vi "PH_BL-Master.PC _6P 4Q Position.vi"(0 "i ref in":refnum<vi>, 2 "6P 4Q Instance":string, 3 "Selector":T1 items=["unknown", "Position I", "Position II", "Position III", "Position IV", "moving"], 4 "no Link":bool, 5 "error in (no error)":errorcluster) -> (14 "i ref out":refnum<vi>, 19 "error out":errorcluster)   [LabVIEW 2014, in "PH_BL-Master.lvlib"]
doc: "This VI writes the incoming information to own attributes."
uses:
  PH_BL-Master.lvlib
  PH_Motion/PH_4_Pos_Selector/PH_4_Pos_Selector.Position Selector.ctl
  PH_Motion/PH_4_Pos_Selector/PH_4_Pos_Selector.lvlib
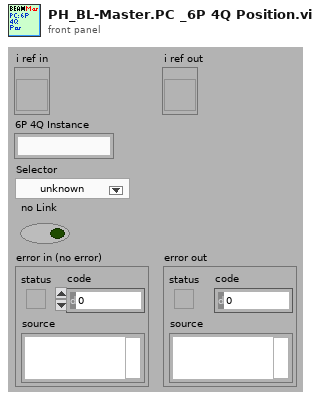
[diagram p1: front panel]
types:
  T1 = typedef "PH_4_Pos_Selector.lvlib/PH_4_Pos_Selector.Position Selector.ctl" = u16
  T2 = typedef "PH_BL-Master.lvlib/PH_BL-Master.i attribute.ctl" = cluster{"Remote controlled":bool, "Boolean Condition Service Subscriber":refnum<vi>[], "Picture Condition Service Subscriber":refnum<vi>[], "R2S":cluster{"GUI Ref":refnum<vi>, "State":bool}, "Vacua":cluster{"GUI Ref":refnum<vi>, "Limit":dbl, "Curr Value":dbl, "in range":bool}[], "O2 Inspection":cluster{"GUI Ref":refnum<vi>, "Concentration":dbl, "State":T3}[], "Boolean Status Service Subscriber":cluster{"GUI Ref":refnum<vi>, "Status":T3, "no Link?":bool, "Status Subscriber Class":T4}[], "Picture Status Service Subscriber":cluster{"GUI Ref":refnum<vi>, "Status":T3, "no Link?":bool, "Status Subscriber Class":T4}[], "6P 4Q Service Subscriber":cluster{"GUI Ref":refnum<vi>, "Selector":T1, "no Link?":bool}[], "Index of latest 6P 4Q changing Instance":i32, "Index of latest Picture Status changing Instance":i32, "Index of latest Boolean Status changing Instance":i32, "Vision ID on same Node":string, "Start Phase over?":bool, "GUI Ref Delete":refnum<vi>}
  T3 = typedef "PH_StatusHandler.lvlib/PH_StatusHandler.Status.ctl" = i16
  T4 = typedef "PH_BL-Master.lvlib/PH_BL-Master.Status Subscriber Class.ctl" = enum16{"unknown", "Switch", "BB", "6P Switch", "Switch GUI", "Switch and 6P State", "Force Sensor"}
  T5 = cluster{"GUI Ref":refnum<vi>, "Selector":T1, "no Link?":bool}[]
  T6 = cluster{"GUI Ref":refnum<vi>, "Selector":T1, "no Link?":bool}
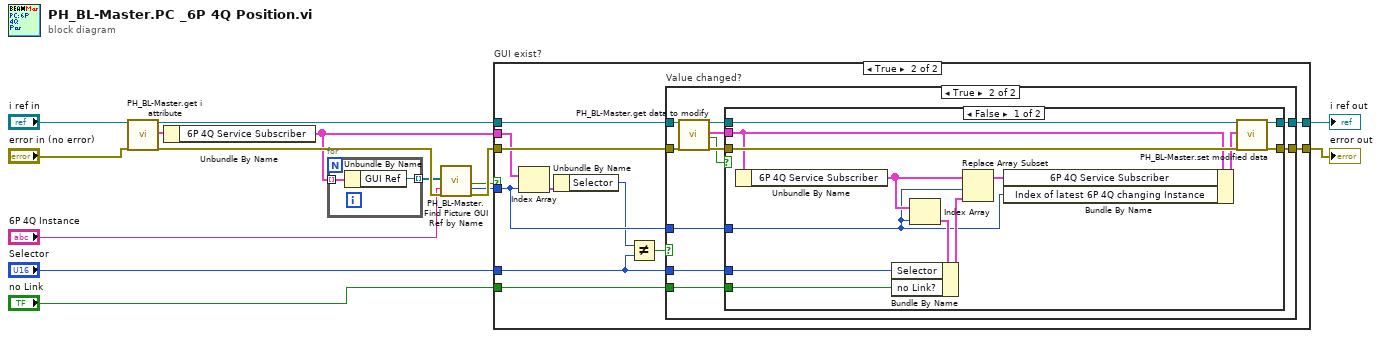
[diagram p0: block diagram]
diagram:
  n1 = call "PH_BL-Master.get i attribute.vi"("i ref in"="i ref in", "error in (no error)"="error in (no error)") -> ("i ref out"=w7:refnum<vi>, "i attribute"=w15:T2, "error out"=w13:errorcluster)  [unwired: 15 in]
  n2 = Unbundle By Name(w15) -> ("6P 4Q Service Subscriber"=w4:T5)
  n3 = for {
    tunnel: w4 -> [w17] mode=indexing
    tunnel: [w16] -> w9 mode=indexing
    n4 = Unbundle By Name(w17) -> ("GUI Ref"=w16:refnum<vi>)
  }
  n5 = call "PH_BL-Master.Find Picture GUI Ref by Name.vi"("Pic Ref Array"=w9, "Label"="6P 4Q Instance", "error in"=w13) -> ("Ref found?"=w1:bool, "index of element"=w3:i32, "error out"=w8:errorcluster)  [unwired: 13 in, 1 out]
  n6 = case "GUI exist?" shown="True" w1 {
    tunnel: [w18 w30] -> w14
    tunnel: [w19 w29] -> w12
    tunnel: w8 -> [w18 w28]
    tunnel: w7 -> [w19 w27]
    tunnel: "no Link" -> [_ w26]
    tunnel: w4 -> [_ w25]
    tunnel: w3 -> [_ w24]
    tunnel: "Selector" -> [_ w21]
    frame False {
    }
    frame True {
      n7 = Index Array(array=w25, index=w24) -> (element=w23:T6)
      n8 = Unbundle By Name(w23) -> ("Selector"=w22:T1)
      n9 = Not Equal?(x=w22, y=w21) -> (x != y?=w20:bool)
      n10 = case "Value changed?" shown="True" w20 {
        tunnel: [w31 w43] -> w30
        tunnel: [w32 w42] -> w29
        tunnel: w28 -> [w31 w41]
        tunnel: w27 -> [w32 w39]
        tunnel: w26 -> [_ w35]
        tunnel: w24 -> [_ w34]
        tunnel: w21 -> [_ w33]
        frame False {
        }
        frame True {
          n11 = call "PH_BL-Master.get data to modify.vi"("i ref in"=w39, "error in (no error)"=w41) -> ("i ref out"=w38:refnum<vi>, "i attribute"=w36:T2, "timed out"=w37:bool, "error out"=w40:errorcluster)  [unwired: 14 in]
          n12 = case shown="False" w37 {
            tunnel: [w56 w57] -> w43
            tunnel: [w55 w58] -> w42
            tunnel: w40 -> [w54 w57]
            tunnel: w38 -> [w53 w58]
            tunnel: w36 -> [w49 _]
            tunnel: w34 -> [w44 _]
            tunnel: w33 -> [w46 _]
            tunnel: w35 -> [w45 _]
            frame False {
              n13 = Unbundle By Name(w49) -> ("6P 4Q Service Subscriber"=w48:T5)
              n14 = Index Array(array=w48, index=w44) -> (element=w51:T6)
              n15 = Bundle By Name(cluster=w51, "Selector"=w46, "no Link?"=w45) -> (w50:T6)
              n16 = Replace Array Subset(array=w48, new element=w50, index=w44) -> (w47:T5)
              n17 = Bundle By Name(cluster=w49, "6P 4Q Service Subscriber"=w47, "Index of latest 6P 4Q changing Instance"=w44) -> (w52:T2)
              n18 = call "PH_BL-Master.set modified data.vi"("i ref in"=w53, "i attribute"=w52, "error in (no error)"=w54) -> ("i ref out"=w55:refnum<vi>, "error out"=w56:errorcluster)  [unwired: 15 in]
            }
            frame True {
            }
          }
        }
      }
    }
  }
  "error out" <- w14
  "i ref out" <- w12
